vi "main3.vi"() -> ()   [LabVIEW 2023]
uses:
  custom_elements/close_button.ctl
  custom_elements/start_button.ctl
  type_defs/data.ctl
  type_defs/states.ctl
  custom_elements/fav_colorctl.ctl
  custom_elements/fav_cartoon.ctl
  custom_elements/fav_places.ctl
  <vilib>/Utility/error.llb/DialogType.ctl
panel:
  in  "Start":T1=TRUE
  out "error constant 2":errorcluster
  in  "error constant":errorcluster
  in  "Close":T2
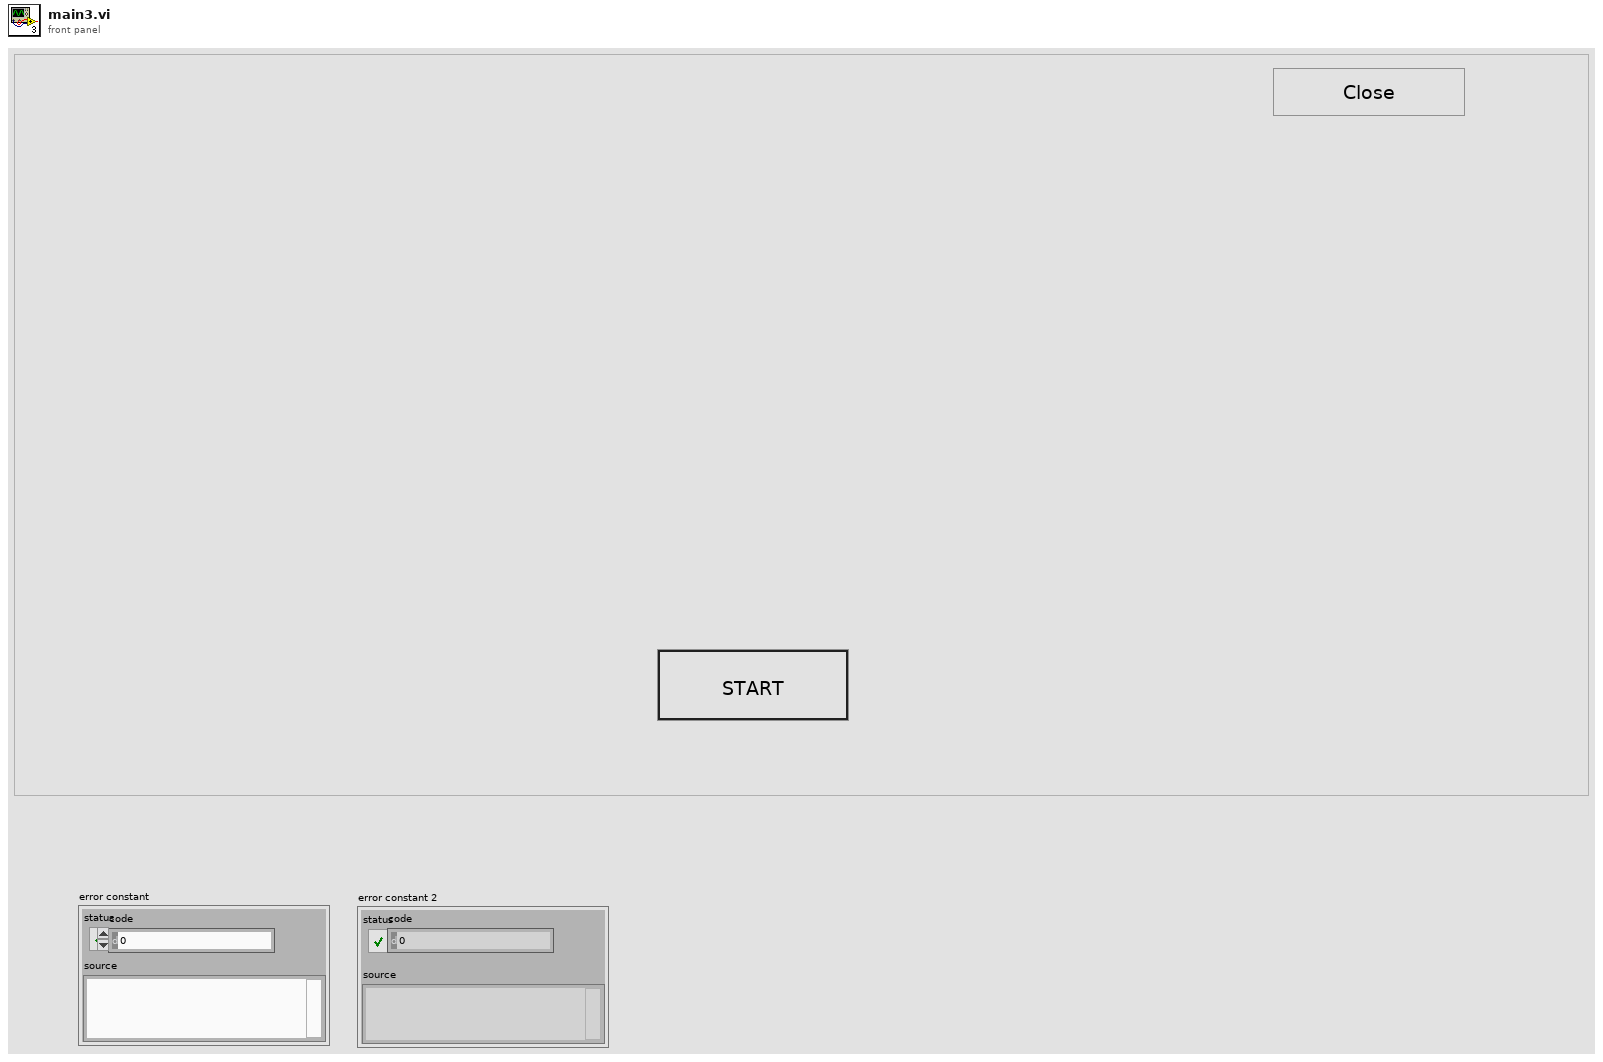
[diagram p1: front panel]
types:
  T1 = typedef "start_button.ctl" = bool
  T2 = typedef "close_button.ctl" = bool
  T3 = typedef "data.ctl" = cluster{"state":T4, "number":dbl, "Name":string, "color":T5, "birthday":timestamp, "cartoon":T6, "place":T7}
  T4 = typedef "states.ctl" = enum16{"idle", "final", "place", "cartoon_character", "colour", "lucky_number", "get_details", "start"}
  T5 = typedef "fav_colorctl.ctl" = enum16{"black", "blue", "green", "red"}
  T6 = typedef "fav_cartoon.ctl" = enum16{"Ben 10", "Shin Chan", "Pokemon", "Tom and Jerry"}
  T7 = typedef "fav_places.ctl" = enum16{"Forest", "Mountain", "Beach", "Home"}
  T8 = typedef "Sound Output Task ID.ctl" = u32
  T9 = typedef "back_button.ctl" = bool
  T10 = typedef "DialogType.ctl" = u16
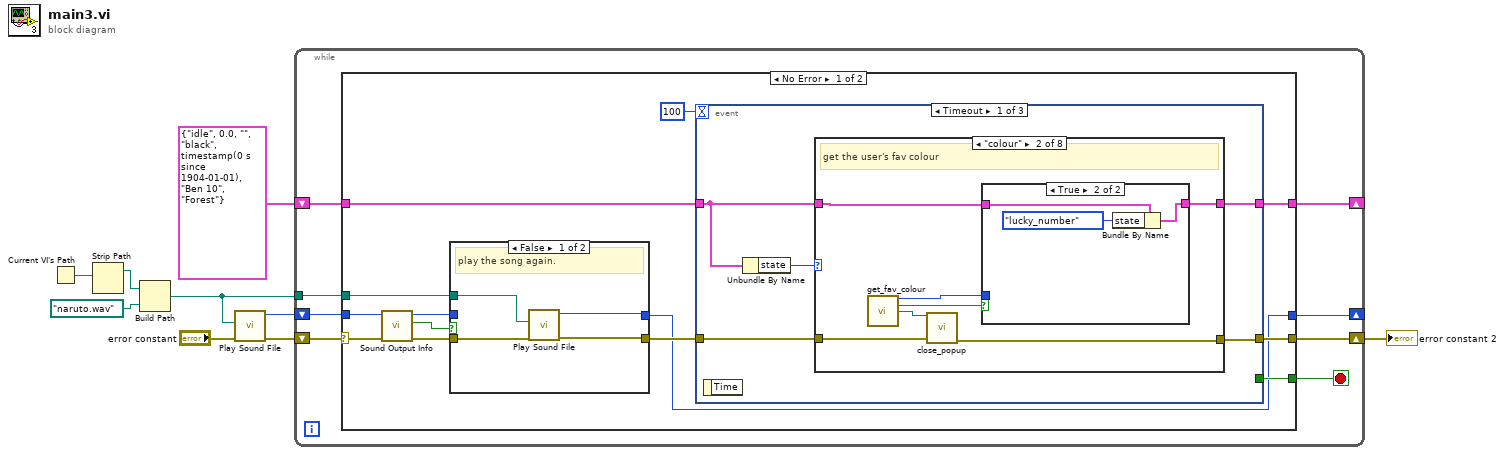
[diagram p0: block diagram]
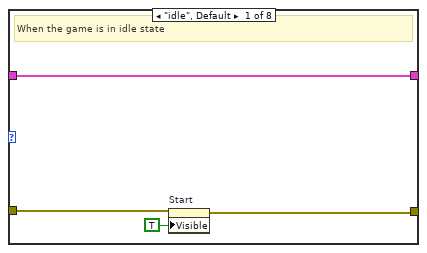
[diagram p3: hidden frame]
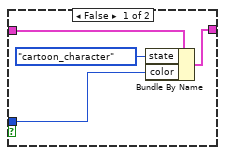
[diagram p4: hidden frame]
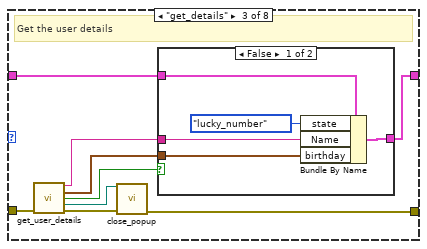
[diagram p5: hidden frame]
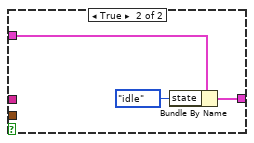
[diagram p6: hidden frame]
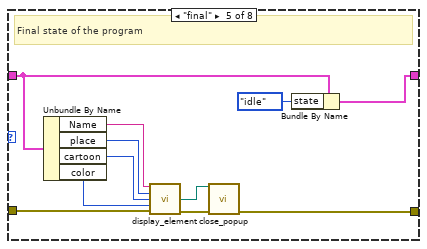
[diagram p8: hidden frame]
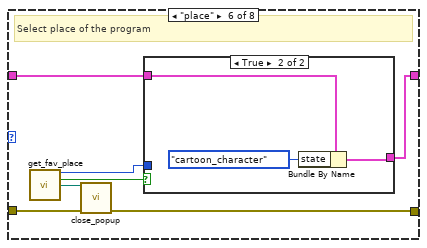
[diagram p9: hidden frame]
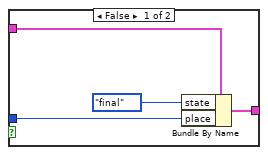
[diagram p10: hidden frame]
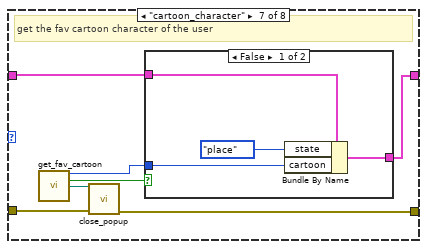
[diagram p11: hidden frame]
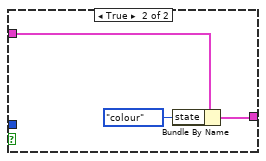
[diagram p12: hidden frame]
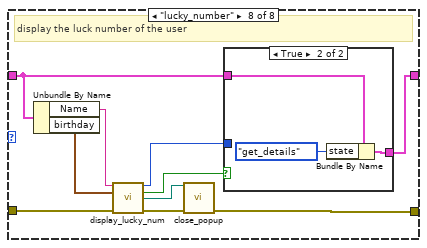
[diagram p13: hidden frame]
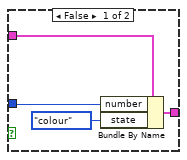
[diagram p14: hidden frame]
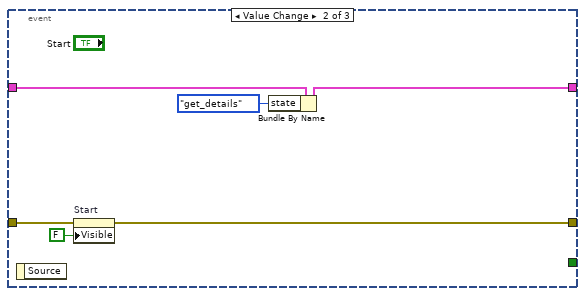
[diagram p15: hidden frame]
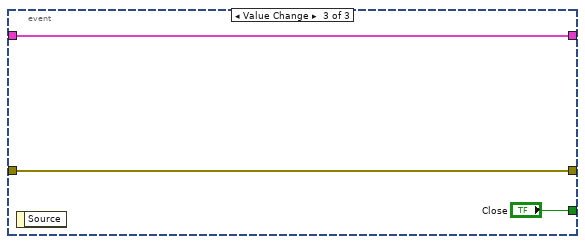
[diagram p16: hidden frame]
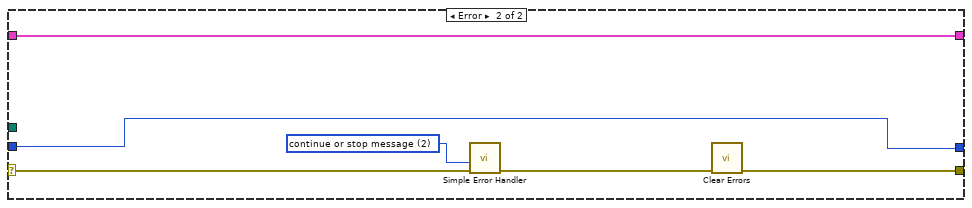
[diagram p17: hidden frame]
diagram:
  n1 = Current VI's Path() -> (path=w4:path)
  n2 = Strip Path(path=w4) -> (stripped path=w3:path)  [unwired: 1 out]
  n3 = Build Path(base path=w3, name or relative path=path "naruto.wav") -> (appended path=w1:path)
  n4 = call <vilib>:"Play Sound File.vi"("error in (no error)"="error constant", "path"=w1) -> ("error out"=w6:errorcluster, "task ID"=w5:T8)  [unwired: 8 in]
  n5 = while {
    shift-right: [w16] -> _
    shift-left: T3 {"state"=enum."idle", "number"=0.0, "Name"="", "color"=enum."black", "birthday"=timestamp(0 s since 1904-01-01), "cartoon"=enum."Ben 10", "place"=enum."Forest"} -> [w15]
    shift-right: [w17] -> w9
    shift-left: w6 -> [w13]
    tunnel: w1 -> [w11]
    shift-right: [w10] -> _
    shift-left: w5 -> [w12]
    stop <- w14 stop-if-true
    n6 = case shown="No Error" w13 {
      selector: w13 -> [w24 w147]
      tunnel: [w29 w144] -> w17
      tunnel: [w28 w149] -> w16
      tunnel: w15 -> [w27 w149]
      tunnel: [w26 _] -> w14
      tunnel: w12 -> [w22 w148]
      tunnel: w11 -> [w20 _]
      tunnel: [w19 w148] -> w10
      frame No Error {
        n7 = call <vilib>:"Sound Output Info.vi"("error in (no error)"=w24, "task ID"=w22) -> ("error out"=w23:errorcluster, "is playing?"=w21:bool, "task ID out"=w18:T8)  [unwired: 6 in, 1 out]
        n8 = case shown="False" w21 {
          tunnel: w23 -> [w34 w36]
          tunnel: [w33 w36] -> w25
          tunnel: w20 -> [w32 _]
          tunnel: [w31 w35] -> w19
          tunnel: w18 -> [_ w35]
          frame False {
            # "play the song again."
            n9 = call <vilib>:"Play Sound File.vi"("error in (no error)"=w34, "path"=w32) -> ("error out"=w33:errorcluster, "task ID"=w31:T8)  [unwired: 8 in]
          }
          frame True {
            # "Continue playing the song"
          }
        }
        n10 = event shown="[0] Timeout" {
          selector: _ -> [_ _ _]
          dyn-events: _ -> [_ _ _]
          timeout: 100 -> [_ _ _]
          tunnel: [w39 w138 w141] -> w29
          tunnel: [w40 w136 w142] -> w28
          tunnel: w27 -> [w37 w137 w142]
          tunnel: [_ _ "Close"] -> w26
          tunnel: w25 -> [w38 w139 w141]
          event Timeout {
            n11 = event-data() -> ()  [unwired: 1 in, 1 out]
            n12 = Unbundle By Name(w37) -> ("state"=w41:T4)
            n13 = case shown="\"colour\"" w41 {
              tunnel: w37 -> [w45 w52 w68 w78 w80 w95 w110 w121]
              tunnel: [w45 w48 w66 w78 w81 w96 w109 w122] -> w40
              tunnel: [w42 w50 w67 w77 w82 w93 w106 w123] -> w39
              tunnel: w38 -> [w44 w47 w61 w77 w85 w94 w107 w124]
              frame "idle", Default {
                # "When the game is in idle state"
                n14 = property on="Start" class="Bool"(error in=w44, "Visible"=TRUE) -> (error out=w42:errorcluster)  [unwired: 1 in, 1 out]
              }
              frame "colour" {
                # "get the user's fav colour"
                n15 = call "get_fav_colour.vi"() -> (4:w51:T5, "Back out"=w46:T9, "path"=w49:path)  [unwired: 13 in]
                n16 = call "close_popup.vi"("path"=w49, "error in (no error)"=w47) -> ("error out"=w50:errorcluster)  [unwired: 13 in]
                n17 = case shown="True" w46 {
                  tunnel: w52 -> [w56 w59]
                  tunnel: w51 -> [w55 _]
                  tunnel: [w54 w58] -> w48
                  frame False {
                    n18 = Bundle By Name(cluster=w56, "state"=states."cartoon_character", "color"=w55) -> (w54:T3)
                  }
                  frame True {
                    n19 = Bundle By Name(cluster=w59, "state"=states."lucky_number") -> (w58:T3)
                  }
                }
              }
              frame "get_details" {
                # "Get the user details"
                n20 = call "get_user_details.vi"("error in (no error)"=w61) -> ("Name 2"=w65:string, "Birthday 2"=w64:timestamp, "Back_out"=w62:T9, "path"=w63:path, "error out"=w60:errorcluster)  [unwired: 10 in]
                n21 = call "close_popup.vi"("path"=w63, "error in (no error)"=w60) -> ("error out"=w67:errorcluster)  [unwired: 13 in]
                n22 = case shown="False" w62 {
                  tunnel: w68 -> [w73 w76]
                  tunnel: [w72 w75] -> w66
                  tunnel: w65 -> [w70 _]
                  tunnel: w64 -> [w69 _]
                  frame False {
                    n23 = Bundle By Name(cluster=w73, "state"=states."lucky_number", "Name"=w70, "birthday"=w69) -> (w72:T3)
                  }
                  frame True {
                    n24 = Bundle By Name(cluster=w76, "state"=states."idle") -> (w75:T3)
                  }
                }
              }
              frame "start" {
                # "Start state of the program"
              }
              frame "final" {
                # "Final state of the program"
                n25 = Unbundle By Name(w80) -> ("Name"=w89:string, "place"=w88:T7, "cartoon"=w87:T6, "color"=w86:T5)
                n26 = call "display_element.vi"("Name"=w89, "place"=w88, "cartoon"=w87, "color"=w86, "error in"=w85) -> ("path"=w84:path, "error out"=w83:errorcluster)  [unwired: 9 in]
                n27 = call "close_popup.vi"("path"=w84, "error in (no error)"=w83) -> ("error out"=w82:errorcluster)  [unwired: 13 in]
                n28 = Bundle By Name(cluster=w80, "state"=states."idle") -> (w81:T3)
              }
              frame "place" {
                # "Select place of the program"
                n29 = call "get_fav_place.vi"() -> ("place"=w92:T7, "Back out"=w90:T9, "path"=w91:path)  [unwired: 13 in]
                n30 = call "close_popup.vi"("path"=w91, "error in (no error)"=w94) -> ("error out"=w93:errorcluster)  [unwired: 13 in]
                n31 = case shown="True" w90 {
                  tunnel: [w99 w103] -> w96
                  tunnel: w95 -> [w98 w102]
                  tunnel: w92 -> [w97 _]
                  frame False {
                    n32 = Bundle By Name(cluster=w98, "state"=states."final", "place"=w97) -> (w99:T3)
                  }
                  frame True {
                    n33 = Bundle By Name(cluster=w102, "state"=states."cartoon_character") -> (w103:T3)
                  }
                }
              }
              frame "cartoon_character" {
                # "get the fav cartoon character of the user"
                n34 = call "get_fav_cartoon.vi"() -> ("Cartoon out"=w105:T6, "Back out"=w104:T9, "path"=w108:path)  [unwired: 13 in]
                n35 = call "close_popup.vi"("path"=w108, "error in (no error)"=w107) -> ("error out"=w106:errorcluster)  [unwired: 13 in]
                n36 = case shown="False" w104 {
                  tunnel: w110 -> [w114 w116]
                  tunnel: [w113 w117] -> w109
                  tunnel: w105 -> [w111 _]
                  frame False {
                    n37 = Bundle By Name(cluster=w114, "state"=states."place", "cartoon"=w111) -> (w113:T3)
                  }
                  frame True {
                    n38 = Bundle By Name(cluster=w116, "state"=states."colour") -> (w117:T3)
                  }
                }
              }
              frame "lucky_number" {
                # "display the luck number of the user"
                n39 = Unbundle By Name(w121) -> ("Name"=w120:string, "birthday"=w119:timestamp)
                n40 = call "display_lucky_num.vi"("Name"=w120, "Birthday"=w119, "error in"=w124) -> ("lucky_num"=w127:i32, "Back 2"=w118:T9, "path"=w126:path, "error out"=w125:errorcluster)  [unwired: 9 in]
                n41 = call "close_popup.vi"("path"=w126, "error in (no error)"=w125) -> ("error out"=w123:errorcluster)  [unwired: 13 in]
                n42 = case shown="True" w118 {
                  tunnel: w127 -> [w131 _]
                  tunnel: [w129 w134] -> w122
                  tunnel: w121 -> [w128 w133]
                  frame False {
                    n43 = Bundle By Name(cluster=w128, "number"=w131, "state"=states."colour") -> (w129:T3)
                  }
                  frame True {
                    n44 = Bundle By Name(cluster=w133, "state"=states."get_details") -> (w134:T3)
                  }
                }
              }
            }
          }
          event Value Change {
            n45 = event-data() -> ()  [unwired: 1 in, 1 out]
            n46 = property on="Start" class="Bool"(error in=w139, "Visible"=FALSE) -> (error out=w138:errorcluster)  [unwired: 1 in, 1 out]
            n47 = Bundle By Name(cluster=w137, "state"=states."get_details") -> (w136:T3)
          }
          event Value Change {
            n48 = event-data() -> ()  [unwired: 1 in, 1 out]
          }
        }
      }
      frame Error {
        w145 = T10 2 items=["no dialog", "OK message", "continue or stop message", "OK message + warnings", "continue/stop + warnings"] ("type of dialog (OK msg:1)")
        n49 = call <vilib>:"Simple Error Handler.vi"("type of dialog (OK msg:1)"=w145, "error in (no error)"=w147) -> ("error out"=w146:errorcluster)  [unwired: 3 in, 4 out]
        n50 = call <vilib>:"Clear Errors.vi"("error in (no error)"=w146) -> ("error out"=w144:errorcluster)  [unwired: 5 in, 1 out]
      }
    }
  }
  "error constant 2" <- w9
